vi "Slope Calibration Waveform.vi"() -> (0 "Slope Calibration Waveform":waveform(dbl)[](array[waveform]))   [LabVIEW 2013]
uses:
  <vilib>/measure/NI_MABase.lvlib
panel:
  in  "Phase Offset":dbl format="%#_13g"
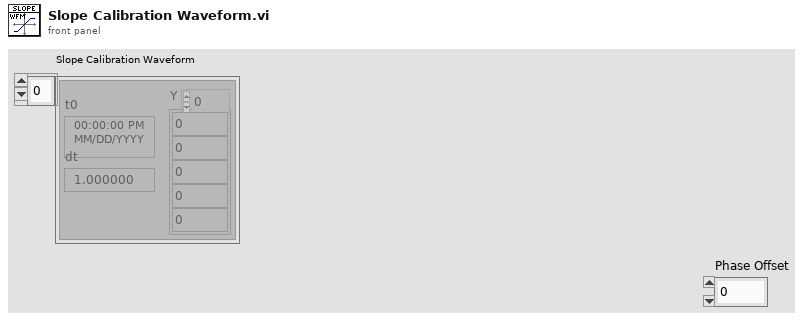
[diagram p1: front panel]
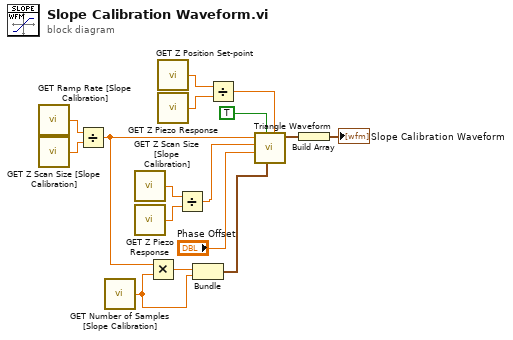
[diagram p0: block diagram]
diagram:
  n1 = call "GET Ramp Rate [Slope Calibration].vi"() -> ("Ramp Rate"=w15:dbl)
  n2 = call "GET Z Scan Size [Slope Calibration].vi"() -> ("Z Scan Size"=w16:dbl)
  n3 = Divide(x=w15, y=w16) -> (x/y=w4:dbl)
  n4 = call "GET Number of Samples [Slope Calibration].vi"() -> ("Number of Samples"=w3:dbl)
  n5 = call "GET Z Scan Size [Slope Calibration].vi"() -> ("Z Scan Size"=w9:dbl)
  n6 = call "GET Z Piezo Response.vi"() -> ("Z Piezo Response"=w10:dbl)
  n7 = Multiply(x=w4, y=w3) -> (x*y=w13:dbl)
  n8 = call "GET Z Position Set-point.vi"() -> ("Z Position Set-point"=w7:dbl)
  n9 = call "GET Z Piezo Response.vi"() -> ("Z Piezo Response"=w6:dbl)
  n10 = Divide(x=w9, y=w10) -> (x/y=w11:dbl)
  n11 = Bundle(w13, "Number of Samples"=w3) -> (w12:cluster{dbl, "Number of Samples":dbl})  [unwired: 1 in]
  n12 = Divide(x=w7, y=w6) -> (x/y=w8:dbl)
  n13 = call <vilib>:"Triangle Waveform.vi"("offset"=w8, "sampling info"=w12, "reset signal"=TRUE, "phase"="Phase Offset", "amplitude"=w11, "frequency"=w4) -> ("signal out"=w2:waveform(dbl))  [unwired: 4 in, 1 out]
  n14 = Build Array(w2) -> (→"Slope Calibration Waveform":waveform(dbl)[])
